vi "WSVCAP SHL Host LL Manage FPGA Top Level Controls Core.vi"(0 "Value In":variant, 1 "FPGA VI Reference (Init Only)":T1, 7 "FPGA Top Level Control":T2=enum."Read Status Flag", 11 "error in (no error)":errorcluster, 12 "Simulate FPGA (Init Only)":bool=TRUE, 13 "Operation":T3) -> (4 "Value Out":variant, 15 "error out":errorcluster)   [LabVIEW 2012]
uses:
  Type Defs/WSVCAP SHL Top Level Control Operation Enum.ctl
  Type Defs/WSVCAP SHL Top Level Control Enum.ctl
  Type Defs/WSVCAP SHL FPGA VI Reference.ctl
  Type Defs/WSVCAP SHL State.ctl
  Type Defs/WSVCAP SHL Transaction Enum.ctl
  <vilib>/Utility/error.llb/Error Cluster From Error Code.vi
  <vilib>/rvi/errors/niLvFpgaAdjustHostInterfaceError.vi
  <vilib>/rvi/interface/nirviReadWriteControl/nirviReadWriteControl.xnode
  FPGA Bitfiles/WSVCAPShell_WiSpryFPGA1_WSVCAPSHLFPGATLT_acCLp6kl0Ls.lvbitx
  NiFpgaLv.dll
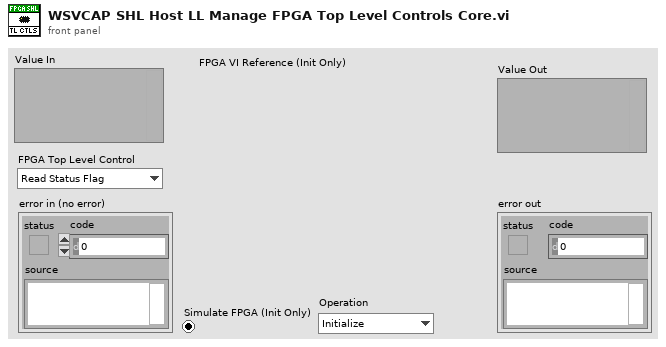
[diagram p1: front panel]
types:
  T1 = typedef "WSVCAP SHL FPGA VI Reference.ctl" = refnum<k20>
  T2 = typedef "WSVCAP SHL Top Level Control Enum.ctl" = enum16{"Start", "Cmd", "Transaction", "Wait Ticks", "Socket Mask", "UUT Set", "Slave Address", "Sub Address", "Bytes to Write", "Bytes to Read", "Write Data", "Write Flag", "Read Data", "Read Flag", "Ack Read", "Read Status Flag", "Ack Read Status", "Status", "Cycle Count", "Stop Cycle", "Exit"}
  T3 = typedef "WSVCAP SHL Top Level Control Operation Enum.ctl" = enum16{"Initialize", "Set Control", "Read Control", "Close"}
  T4 = typedef "WSVCAP SHL State.ctl" = enum8{"Idle", "Transfer Data"}
  T5 = typedef "WSVCAP SHL Transaction Enum.ctl" = enum16{"I2C-Read Data", "I2C-Write Data", "RFFE-Ext Write", "RFFE-Ext Read"}
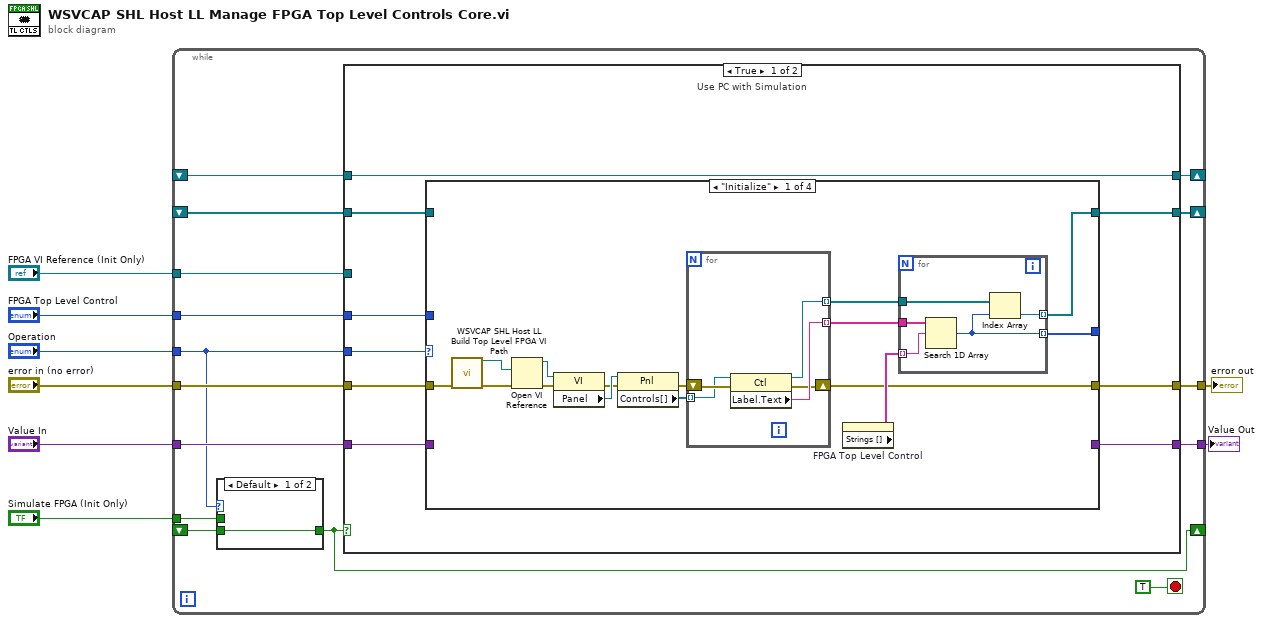
[diagram p0: block diagram]
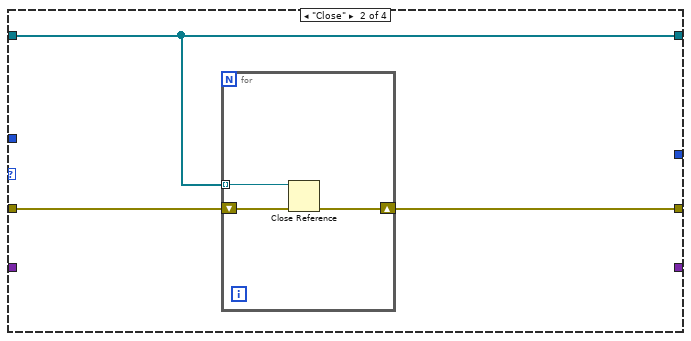
[diagram p2: hidden frame]
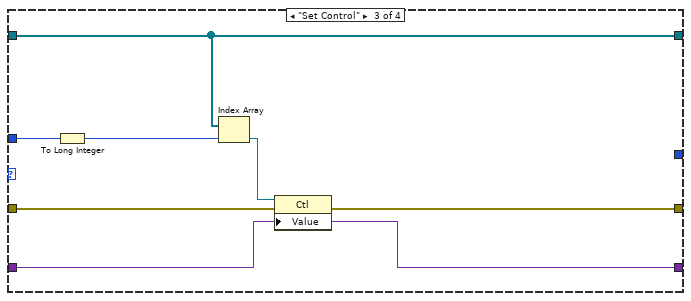
[diagram p3: hidden frame]
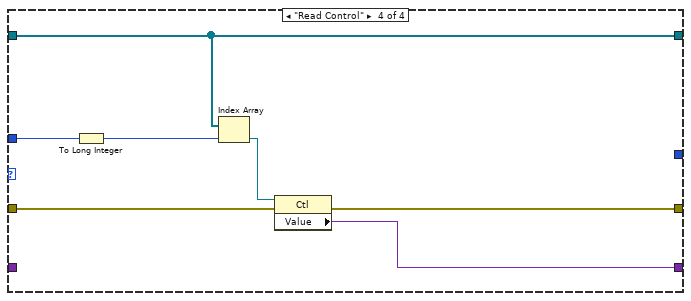
[diagram p4: hidden frame]
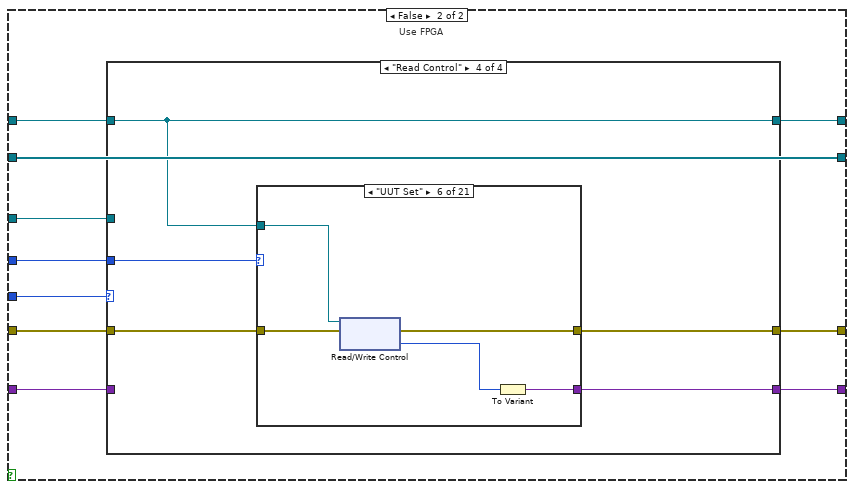
[diagram p5: hidden frame]
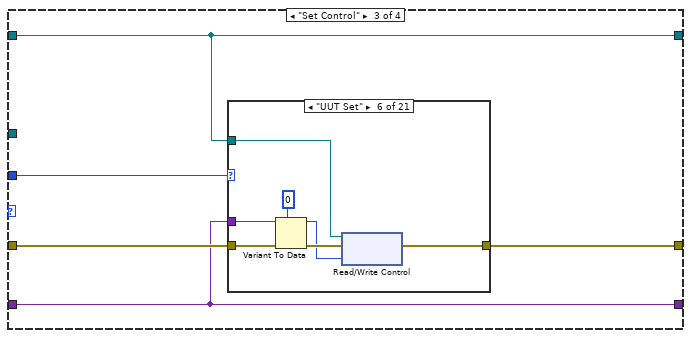
[diagram p8: hidden frame]
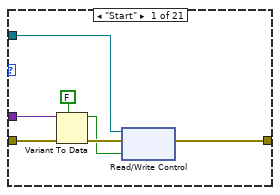
[diagram p9: hidden frame]
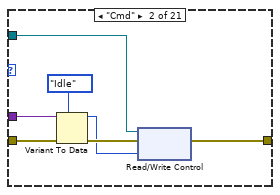
[diagram p10: hidden frame]
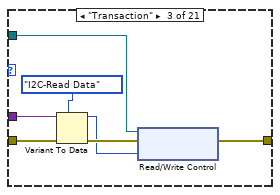
[diagram p11: hidden frame]
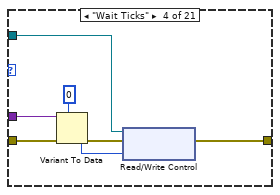
[diagram p12: hidden frame]
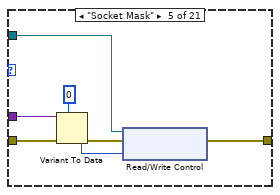
[diagram p13: hidden frame]
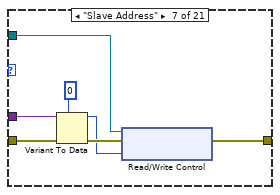
[diagram p14: hidden frame]
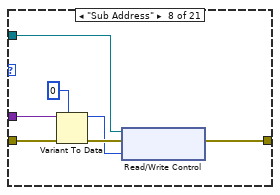
[diagram p15: hidden frame]
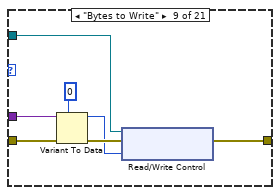
[diagram p16: hidden frame]
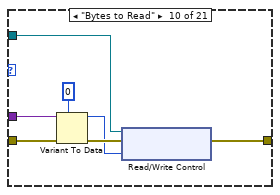
[diagram p17: hidden frame]
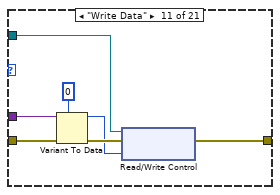
[diagram p18: hidden frame]
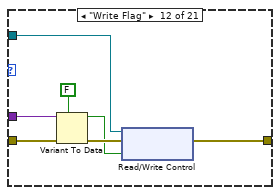
[diagram p19: hidden frame]
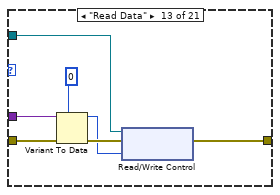
[diagram p20: hidden frame]
diagram:
  n1 = while {
    tunnel: [w23] -> w8
    tunnel: "error in (no error)" -> [w22]
    tunnel: [w21] -> w6
    tunnel: "Value In" -> [w20]
    tunnel: "FPGA Top Level Control" -> [w19]
    tunnel: "FPGA VI Reference (Init Only)" -> [w18]
    tunnel: "Operation" -> [w17]
    tunnel: "Simulate FPGA (Init Only)" -> [w11]
    shift-right: [w12] -> _
    shift-left: _ -> [w13]
    shift-right: [w15] -> _
    shift-left: _ -> [w14]
    shift-right: [w9] -> _
    shift-left: _ -> [w10]
    stop <- TRUE stop-if-true
    n2 = case shown="Default" w17 {
      tunnel: [w353 w354] -> w9
      tunnel: w11 -> [_ w354]
      tunnel: w10 -> [w353 _]
      frame Default {
      }
      frame "Initialize" {
        # "Load Sim Mode"
      }
    }
    n3 = case shown="True" w9 {
      tunnel: w17 -> [w32 w87]
      tunnel: [w31 w86] -> w23
      tunnel: w22 -> [w30 w85]
      tunnel: [w29 w84] -> w21
      tunnel: w20 -> [w28 w83]
      tunnel: w19 -> [w27 w82]
      tunnel: w18 -> [_ w81]
      tunnel: [w26 w78] -> w15
      tunnel: w14 -> [w25 w78]
      tunnel: w13 -> [w24 w80]
      tunnel: [w24 w79] -> w12
      frame True {
        # "Use PC with Simulation"
        n4 = case shown="\"Initialize\"" w32 {
          tunnel: [w41 w60 w70 w77] -> w26
          tunnel: w25 -> [_ w60 w70 w77]
          tunnel: [w37 w59 w67 w74] -> w31
          tunnel: w30 -> [w35 w58 w68 w75]
          tunnel: [_ _ w66 w73] -> w29
          tunnel: w28 -> [_ _ w66 _]
          tunnel: w27 -> [_ _ w65 w72]
          tunnel: [w36 _ _ _] -> _
          frame "Initialize" {
            n5 = call "WSVCAP SHL Host LL Build Top Level FPGA VI Path.vi"("Error In (no error)"=w35) -> ("Top Level FPGA VI Path"=w33:path, "Error Out"=w34:errorcluster)  [unwired: 13 in]
            n6 = Open VI Reference(vi path=w33, error in (no error)=w34) -> (vi reference=w47:refnum<vi>, error out=w40:errorcluster)  [unwired: 4 in]
            n7 = property class="VI"(reference=w47, error in=w40) -> (error out=w39:errorcluster, "Panel"=w46:refnum<vi>)  [unwired: 1 out]
            n8 = property class="Pnl"(reference=w46, error in=w39) -> (error out=w38:errorcluster, "Controls[]"=w45:refnum<vi>[])  [unwired: 1 out]
            n9 = for {
              tunnel: w45 -> [w53] mode=indexing
              tunnel: [w57] -> w42 mode=indexing
              tunnel: [w56] -> w44 mode=indexing
              shift-right: [w54] -> w37
              shift-left: w38 -> [w55]
              n10 = property class="Ctl"(reference=w53, error in=w55) -> (reference out=w57:refnum<vi>, error out=w54:errorcluster, "Label.Text"=w56:string)
            }
            n11 = property on="FPGA Top Level Control" class="Enum (strict)"() -> ("Strings []"=w43:string[])  [unwired: 2 in, 2 out]
            n12 = for {
              tunnel: w44 -> [w52]
              tunnel: w43 -> [w51] mode=indexing
              tunnel: w42 -> [w50]
              tunnel: [w49] -> w41 mode=indexing
              tunnel: [w48] -> w36 mode=indexing
              n13 = Search 1D Array(1D array=w52, element=w51) -> (index of element=w48:i32)  [unwired: 1 in]
              n14 = Index Array(array=w50, index=w48) -> (element=w49:refnum<vi>)
            }
          }
          frame "Close" {
            n15 = for {
              tunnel: w60 -> [w63] mode=indexing
              shift-right: [w62] -> w59
              shift-left: w58 -> [w61]
              n16 = Close Reference(reference=w63, error in (no error)=w61) -> (error out=w62:errorcluster)
            }
          }
          frame "Set Control" {
            n17 = To Long Integer(number=w65) -> (32bit integer=w64:i32)
            n18 = Index Array(array=w70, index=w64) -> (element=w69:refnum<vi>)
            n19 = property class="Ctl"(reference=w69, error in=w68, "Value"=w66) -> (error out=w67:errorcluster)  [unwired: 1 out]
          }
          frame "Read Control" {
            n20 = To Long Integer(number=w72) -> (32bit integer=w71:i32)
            n21 = Index Array(array=w77, index=w71) -> (element=w76:refnum<vi>)
            n22 = property class="Ctl"(reference=w76, error in=w75) -> (error out=w74:errorcluster, "Value"=w73:variant)  [unwired: 1 out]
          }
        }
      }
      frame False {
        # "Use FPGA"
        n23 = case shown="\"Read Control\"" w87 {
          tunnel: [w88 w91 w95 w246] -> w86
          tunnel: w85 -> [w88 w91 w96 w247]
          tunnel: [_ _ w93 w243] -> w84
          tunnel: w83 -> [_ _ w93 _]
          tunnel: w82 -> [_ _ w94 w245]
          tunnel: [w89 w90 w92 w244] -> w79
          tunnel: w80 -> [_ w90 w92 w244]
          tunnel: w81 -> [w89 _ _ _]
          frame "Initialize" {
          }
          frame "Close" {
          }
          frame "Set Control" {
            n24 = case shown="\"UUT Set\"" w94 {
              tunnel: w92 -> [w103 w110 w117 w124 w131 w138 w145 w152 w159 w166 w173 w180 w187 w194 w201 w208 w215 w222 w228 w235 w242]
              tunnel: w96 -> [w102 w109 w116 w123 w130 w137 w144 w151 w158 w165 w172 w179 w186 w193 w200 w207 w214 w221 w227 w234 w241]
              tunnel: [w100 w107 w114 w121 w128 w135 w142 w149 w156 w163 w170 w177 w184 w191 w198 w205 w212 w219 w225 w232 w239] -> w95
              tunnel: w93 -> [w99 w106 w113 w120 w127 w134 w141 w148 w155 w162 w169 w176 w183 w190 w197 w204 w211 w218 w224 w231 w238]
              frame "Start" {
                n25 = Variant To Data(error in=w102, type=FALSE ("SPI_CPOL"), Variant=w99) -> (data=w98:bool, error out=w101:errorcluster)
                n26 = xnode "Read/Write Control"("FPGA VI Reference In"=w103, "error in"=w101, "Start"=w98) -> ("error out"=w100:errorcluster)  [unwired: 1 out]
              }
              frame "Cmd" {
                n27 = Variant To Data(error in=w109, type=WSVCAP_SHL_State."Idle" ("SPI_Cmd"), Variant=w106) -> (data=w104:T4, error out=w108:errorcluster)
                n28 = xnode "Read/Write Control"("FPGA VI Reference In"=w110, "error in"=w108, "Cmd"=w104) -> ("error out"=w107:errorcluster)  [unwired: 1 out]
              }
              frame "Transaction" {
                n29 = Variant To Data(error in=w116, type=WSVCAP_SHL_Transaction_Enum."I2C-Read Data" ("Transaction"), Variant=w113) -> (data=w111:T5, error out=w115:errorcluster)
                n30 = xnode "Read/Write Control"("FPGA VI Reference In"=w117, "error in"=w115, "Transaction"=w111) -> ("error out"=w114:errorcluster)  [unwired: 1 out]
              }
              frame "Wait Ticks" {
                n31 = Variant To Data(error in=w123, type=u32 0 ("I2C_Clock Divider"), Variant=w120) -> (data=w119:u32, error out=w122:errorcluster)
                n32 = xnode "Read/Write Control"("FPGA VI Reference In"=w124, "error in"=w122, "Wait Ticks"=w119) -> ("error out"=w121:errorcluster)  [unwired: 1 out]
              }
              frame "Socket Mask" {
                n33 = Variant To Data(error in=w130, type=u64 0 ("I2C_Clock Divider"), Variant=w127) -> (data=w126:u64, error out=w129:errorcluster)
                n34 = xnode "Read/Write Control"("FPGA VI Reference In"=w131, "error in"=w129, "Socket Mask"=w126) -> ("error out"=w128:errorcluster)  [unwired: 1 out]
              }
              frame "UUT Set" {
                n35 = Variant To Data(error in=w137, type=u8 0 ("I2C_Clock Divider"), Variant=w134) -> (data=w132:u8, error out=w136:errorcluster)
                n36 = xnode "Read/Write Control"("FPGA VI Reference In"=w138, "error in"=w136, "UUT Set"=w132) -> ("error out"=w135:errorcluster)  [unwired: 1 out]
              }
              frame "Slave Address" {
                n37 = Variant To Data(error in=w144, type=u8 0 ("I2C_Slave Address"), Variant=w141) -> (data=w140:u8, error out=w143:errorcluster)
                n38 = xnode "Read/Write Control"("FPGA VI Reference In"=w145, "error in"=w143, "Slave Address"=w140) -> ("error out"=w142:errorcluster)  [unwired: 1 out]
              }
              frame "Sub Address" {
                n39 = Variant To Data(error in=w151, type=u8 0 ("SPI_CS"), Variant=w148) -> (data=w146:u8, error out=w150:errorcluster)
                n40 = xnode "Read/Write Control"("FPGA VI Reference In"=w152, "error in"=w150, "Sub Address"=w146) -> ("error out"=w149:errorcluster)  [unwired: 1 out]
              }
              frame "Bytes to Write" {
                n41 = Variant To Data(error in=w158, type=u8 0 ("SPI_Clock Divider"), Variant=w155) -> (data=w154:u8, error out=w157:errorcluster)
                n42 = xnode "Read/Write Control"("FPGA VI Reference In"=w159, "error in"=w157, "Bytes to Write"=w154) -> ("error out"=w156:errorcluster)  [unwired: 1 out]
              }
              frame "Bytes to Read" {
                n43 = Variant To Data(error in=w165, type=u8 0 ("SPI_Total Bytes"), Variant=w162) -> (data=w161:u8, error out=w164:errorcluster)
                n44 = xnode "Read/Write Control"("FPGA VI Reference In"=w166, "error in"=w164, "Bytes to Read"=w161) -> ("error out"=w163:errorcluster)  [unwired: 1 out]
              }
              frame "Write Data" {
                n45 = Variant To Data(error in=w172, type=u64 0 ("SPI_Total Bytes"), Variant=w169) -> (data=w168:u64, error out=w171:errorcluster)
                n46 = xnode "Read/Write Control"("FPGA VI Reference In"=w173, "error in"=w171, "Write Data"=w168) -> ("error out"=w170:errorcluster)  [unwired: 1 out]
              }
              frame "Write Flag" {
                n47 = Variant To Data(error in=w179, type=FALSE, Variant=w176) -> (data=w175:bool, error out=w178:errorcluster)
                n48 = xnode "Read/Write Control"("FPGA VI Reference In"=w180, "error in"=w178, "Write Flag"=w175) -> ("error out"=w177:errorcluster)  [unwired: 1 out]
              }
              frame "Read Data" {
                n49 = Variant To Data(error in=w186, type=u64 0 ("I2C_Read Data"), Variant=w183) -> (data=w181:u64, error out=w185:errorcluster)
                n50 = xnode "Read/Write Control"("FPGA VI Reference In"=w187, "error in"=w185, "Read Data"=w181) -> ("error out"=w184:errorcluster)  [unwired: 1 out]
              }
              frame "Read Flag" {
                n51 = Variant To Data(error in=w193, type=FALSE ("SPI_CPOL"), Variant=w190) -> (data=w188:bool, error out=w192:errorcluster)
                n52 = xnode "Read/Write Control"("FPGA VI Reference In"=w194, "error in"=w192, "Read Flag"=w188) -> ("error out"=w191:errorcluster)  [unwired: 1 out]
              }
              frame "Ack Read" {
                n53 = Variant To Data(error in=w200, type=FALSE ("SPI_CPOL"), Variant=w197) -> (data=w196:bool, error out=w199:errorcluster)
                n54 = xnode "Read/Write Control"("FPGA VI Reference In"=w201, "error in"=w199, "Ack Read"=w196) -> ("error out"=w198:errorcluster)  [unwired: 1 out]
              }
              frame "Read Status Flag" {
                n55 = Variant To Data(error in=w207, type=FALSE ("SPI_CPOL"), Variant=w204) -> (data=w203:bool, error out=w206:errorcluster)
                n56 = xnode "Read/Write Control"("FPGA VI Reference In"=w208, "error in"=w206, "Read Status Flag"=w203) -> ("error out"=w205:errorcluster)  [unwired: 1 out]
              }
              frame "Ack Read Status" {
                n57 = Variant To Data(error in=w214, type=FALSE ("SPI_CPOL"), Variant=w211) -> (data=w210:bool, error out=w213:errorcluster)
                n58 = xnode "Read/Write Control"("FPGA VI Reference In"=w215, "error in"=w213, "Ack Read Status"=w210) -> ("error out"=w212:errorcluster)  [unwired: 1 out]
              }
              frame "Status" {
                n59 = Variant To Data(error in=w221, type=0 ("I2C_Status"), Variant=w218) -> (data=w216:i32, error out=w220:errorcluster)
                n60 = xnode "Read/Write Control"("FPGA VI Reference In"=w222, "error in"=w220, "Status"=w216) -> ("error out"=w219:errorcluster)  [unwired: 1 out]
              }
              frame "Cycle Count" {
                w223 = u64 0 ("Cycle Count")
                n61 = Variant To Data(error in=w227, type=w223, Variant=w224) -> (error out=w226:errorcluster)  [unwired: 1 out]
                n62 = xnode "Read/Write Control"("FPGA VI Reference In"=w228, "error in"=w226, "Cycle Count"=w223) -> ("error out"=w225:errorcluster)  [unwired: 1 out]
              }
              frame "Stop Cycle" {
                n63 = Variant To Data(error in=w234, type=FALSE ("SPI_CPOL"), Variant=w231) -> (data=w230:bool, error out=w233:errorcluster)
                n64 = xnode "Read/Write Control"("FPGA VI Reference In"=w235, "error in"=w233, "Stop Cycle"=w230) -> ("error out"=w232:errorcluster)  [unwired: 1 out]
              }
              frame "Exit" {
                n65 = Variant To Data(error in=w241, type=FALSE ("I2C_Exit"), Variant=w238) -> (data=w237:bool, error out=w240:errorcluster)
                n66 = xnode "Read/Write Control"("FPGA VI Reference In"=w242, "error in"=w240, "Exit"=w237) -> ("error out"=w239:errorcluster)  [unwired: 1 out]
              }
            }
          }
          frame "Read Control" {
            n67 = case shown="\"UUT Set\"" w245 {
              tunnel: w244 -> [w252 w257 w262 w267 w272 w277 w282 w287 w292 w297 w302 w307 w312 w317 w322 w327 w332 w337 w342 w347 w352]
              tunnel: w247 -> [w250 w255 w260 w263 w268 w273 w278 w283 w290 w295 w299 w305 w310 w315 w320 w325 w330 w335 w340 w345 w350]
              tunnel: [w251 w256 w261 w266 w271 w276 w281 w286 w291 w296 w301 w306 w311 w316 w321 w326 w331 w336 w341 w346 w351] -> w246
              tunnel: [w248 w253 w259 w264 w269 w274 w279 w284 w288 w293 w298 w303 w308 w313 w318 w323 w328 w333 w338 w343 w348] -> w243
              frame "Start" {
                n68 = xnode "Read/Write Control"("FPGA VI Reference In"=w252, "error in"=w250) -> ("error out"=w251:errorcluster, "Start"=w249:bool)  [unwired: 1 out]
                n69 = To Variant(anything=w249) -> (Variant=w248:variant)
              }
              frame "Cmd" {
                n70 = xnode "Read/Write Control"("FPGA VI Reference In"=w257, "error in"=w255) -> ("error out"=w256:errorcluster, "Cmd"=w254:T4)  [unwired: 1 out]
                n71 = To Variant(anything=w254) -> (Variant=w253:variant)
              }
              frame "Transaction" {
                n72 = xnode "Read/Write Control"("FPGA VI Reference In"=w262, "error in"=w260) -> ("error out"=w261:errorcluster, "Transaction"=w258:T5)  [unwired: 1 out]
                n73 = To Variant(anything=w258) -> (Variant=w259:variant)
              }
              frame "Wait Ticks" {
                n74 = xnode "Read/Write Control"("FPGA VI Reference In"=w267, "error in"=w263) -> ("error out"=w266:errorcluster, "Wait Ticks"=w265:u32)  [unwired: 1 out]
                n75 = To Variant(anything=w265) -> (Variant=w264:variant)
              }
              frame "Socket Mask" {
                n76 = xnode "Read/Write Control"("FPGA VI Reference In"=w272, "error in"=w268) -> ("error out"=w271:errorcluster, "Socket Mask"=w270:u64)  [unwired: 1 out]
                n77 = To Variant(anything=w270) -> (Variant=w269:variant)
              }
              frame "UUT Set" {
                n78 = xnode "Read/Write Control"("FPGA VI Reference In"=w277, "error in"=w273) -> ("error out"=w276:errorcluster, "UUT Set"=w275:u8)  [unwired: 1 out]
                n79 = To Variant(anything=w275) -> (Variant=w274:variant)
              }
              frame "Cycle Count" {
                n80 = xnode "Read/Write Control"("FPGA VI Reference In"=w282, "error in"=w278) -> ("error out"=w281:errorcluster, "Cycle Count"=w280:u64)  [unwired: 1 out]
                n81 = To Variant(anything=w280) -> (Variant=w279:variant)
              }
              frame "Stop Cycle" {
                n82 = xnode "Read/Write Control"("FPGA VI Reference In"=w287, "error in"=w283) -> ("error out"=w286:errorcluster, "Stop Cycle"=w285:bool)  [unwired: 1 out]
                n83 = To Variant(anything=w285) -> (Variant=w284:variant)
              }
              frame "Slave Address" {
                n84 = xnode "Read/Write Control"("FPGA VI Reference In"=w292, "error in"=w290) -> ("error out"=w291:errorcluster, "Slave Address"=w289:u8)  [unwired: 1 out]
                n85 = To Variant(anything=w289) -> (Variant=w288:variant)
              }
              frame "Sub Address" {
                n86 = xnode "Read/Write Control"("FPGA VI Reference In"=w297, "error in"=w295) -> ("error out"=w296:errorcluster, "Sub Address"=w294:u8)  [unwired: 1 out]
                n87 = To Variant(anything=w294) -> (Variant=w293:variant)
              }
              frame "Bytes to Write" {
                n88 = xnode "Read/Write Control"("FPGA VI Reference In"=w302, "error in"=w299) -> ("error out"=w301:errorcluster, "Bytes to Write"=w300:u8)  [unwired: 1 out]
                n89 = To Variant(anything=w300) -> (Variant=w298:variant)
              }
              frame "Bytes to Read" {
                n90 = xnode "Read/Write Control"("FPGA VI Reference In"=w307, "error in"=w305) -> ("error out"=w306:errorcluster, "Bytes to Read"=w304:u8)  [unwired: 1 out]
                n91 = To Variant(anything=w304) -> (Variant=w303:variant)
              }
              frame "Write Data" {
                n92 = xnode "Read/Write Control"("FPGA VI Reference In"=w312, "error in"=w310) -> ("error out"=w311:errorcluster, "Write Data"=w309:u64)  [unwired: 1 out]
                n93 = To Variant(anything=w309) -> (Variant=w308:variant)
              }
              frame "Write Flag" {
                n94 = xnode "Read/Write Control"("FPGA VI Reference In"=w317, "error in"=w315) -> ("error out"=w316:errorcluster, "Write Flag"=w314:bool)  [unwired: 1 out]
                n95 = To Variant(anything=w314) -> (Variant=w313:variant)
              }
              frame "Read Data" {
                n96 = xnode "Read/Write Control"("FPGA VI Reference In"=w322, "error in"=w320) -> ("error out"=w321:errorcluster, "Read Data"=w319:u64)  [unwired: 1 out]
                n97 = To Variant(anything=w319) -> (Variant=w318:variant)
              }
              frame "Read Flag" {
                n98 = xnode "Read/Write Control"("FPGA VI Reference In"=w327, "error in"=w325) -> ("error out"=w326:errorcluster, "Read Flag"=w324:bool)  [unwired: 1 out]
                n99 = To Variant(anything=w324) -> (Variant=w323:variant)
              }
              frame "Ack Read" {
                n100 = xnode "Read/Write Control"("FPGA VI Reference In"=w332, "error in"=w330) -> ("error out"=w331:errorcluster, "Ack Read"=w329:bool)  [unwired: 1 out]
                n101 = To Variant(anything=w329) -> (Variant=w328:variant)
              }
              frame "Read Status Flag" {
                n102 = xnode "Read/Write Control"("FPGA VI Reference In"=w337, "error in"=w335) -> ("error out"=w336:errorcluster, "Read Status Flag"=w334:bool)  [unwired: 1 out]
                n103 = To Variant(anything=w334) -> (Variant=w333:variant)
              }
              frame "Ack Read Status" {
                n104 = xnode "Read/Write Control"("FPGA VI Reference In"=w342, "error in"=w340) -> ("error out"=w341:errorcluster, "Ack Read Status"=w339:bool)  [unwired: 1 out]
                n105 = To Variant(anything=w339) -> (Variant=w338:variant)
              }
              frame "Status" {
                n106 = xnode "Read/Write Control"("FPGA VI Reference In"=w347, "error in"=w345) -> ("error out"=w346:errorcluster, "Status"=w344:i32)  [unwired: 1 out]
                n107 = To Variant(anything=w344) -> (Variant=w343:variant)
              }
              frame "Exit" {
                n108 = xnode "Read/Write Control"("FPGA VI Reference In"=w352, "error in"=w350) -> ("error out"=w351:errorcluster, "Exit"=w349:bool)  [unwired: 1 out]
                n109 = To Variant(anything=w349) -> (Variant=w348:variant)
              }
            }
          }
        }
      }
    }
  }
  "error out" <- w8
  "Value Out" <- w6
